vi "Get Paragraphs.vi"(8 "error in (no error)":errorcluster, 11 "xwpfTable in":refnum<class "xwpfTable.lvclass">) -> (0 "error out":errorcluster, 2 "Paragraphs":refnum<class "xwpfParagraph.lvclass">[](array[class]), 3 "xwpfTable out":refnum<class "xwpfTable.lvclass">)   [LabVIEW 2017, in "Word_Specific.lvlib" / "xwpfTable.lvclass"]
uses:
  xwpfTable.lvclass
  xwpfParagraph/xwpfParagraph.lvclass
  xwpfTable.lvclass/xwpfTable.ctl
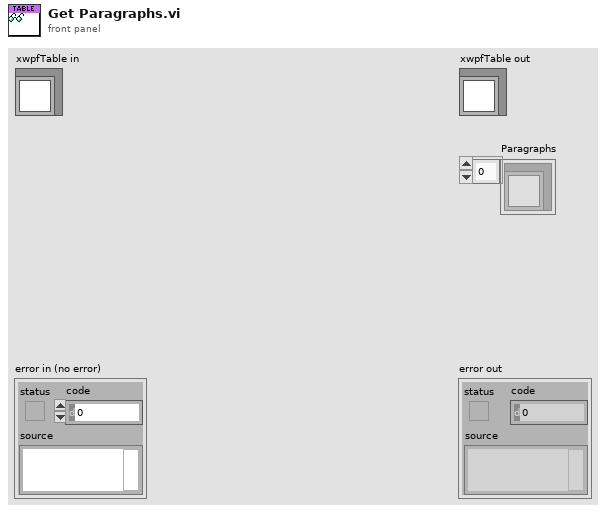
[diagram p1: front panel]
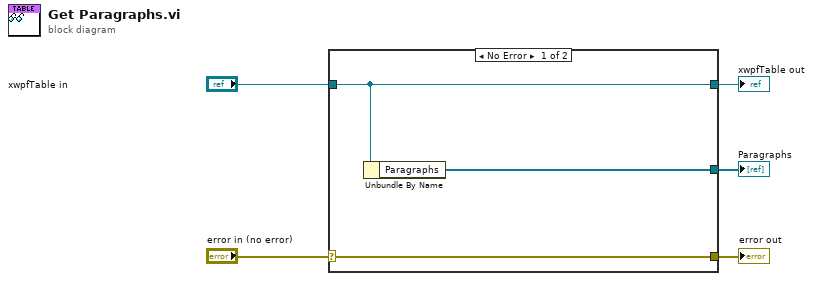
[diagram p0: block diagram]
diagram:
  n1 = case shown="No Error" "error in (no error)" {
    selector: "error in (no error)" -> [w8 w9]
    tunnel: [w8 w9] -> w4
    tunnel: [w7 w10] -> w2
    tunnel: "xwpfTable in" -> [w7 w10]
    tunnel: [w6 _] -> w1
    frame No Error {
      n2 = Unbundle By Name(w7) -> ("Paragraphs"=w6:refnum<class "xwpfParagraph.lvclass">[])
    }
    frame Error {
    }
  }
  "error out" <- w4
  "xwpfTable out" <- w2
  "Paragraphs" <- w1
